vi "Day12-validate_path_2.vi"(11 "Path":string[](array[string])) -> (1 "invalid?":bool, 2 "finshed?":bool, 3 "Path out":string[](array[string]))   [LabVIEW 2021]
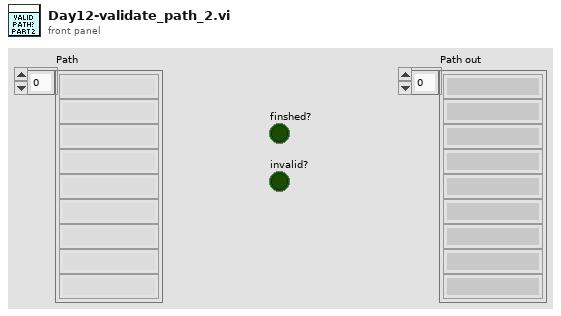
[diagram p1: front panel]
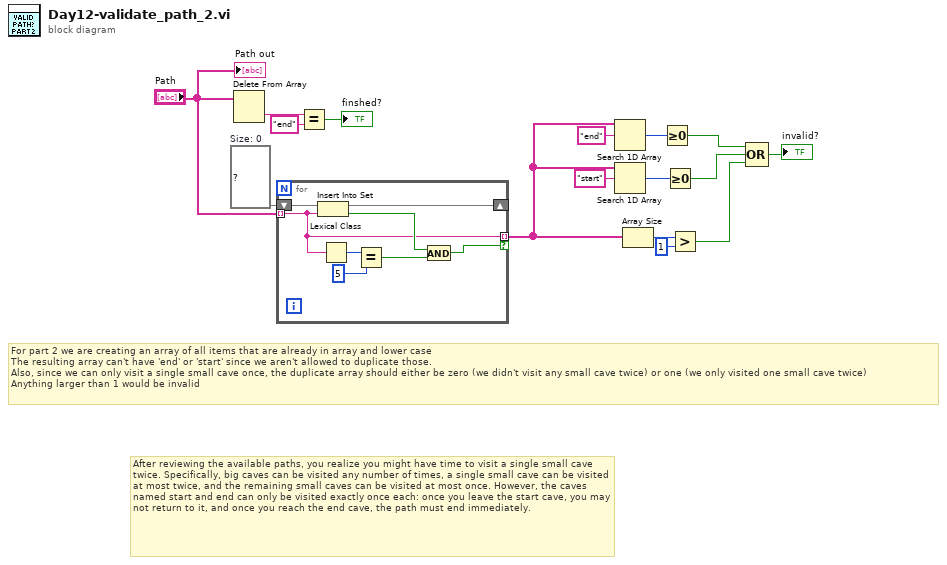
[diagram p0: block diagram]
diagram:
  w13 = set{string} {}  # Size: 0
  # "After reviewing the available paths, you realize you might have time to visit a single small cave twice. Specifically, big caves can be visited any number of times, a single small cave can be visited at most twice, and the remaining small caves can be visited at most once. However, the caves named start and end can only be visited exactly once each: once you leave the start cave, you may not return to it, and once you reach the end cave, the path must end immediately."
  # "For part 2 we are creating an array of all items that are already in array and lower case\nThe resulting array can't have 'end' or 'start' since we aren't allowed to duplicate those.\nAlso, since we can only visit a single small cave once, the duplicate array should either be zero (we didn't visit any small cave twice) or one (we only visited one small cave twice)\nAnything larger than 1 would be invalid"
  n1 = Delete From Array(array="Path") -> (deleted portion=w16:string)  [unwired: 2 in, 1 out]
  n2 = for {
    tunnel: "Path" -> [w18] mode=indexing
    shift-right: [w24] -> _
    shift-left: w13 -> [w23]
    tunnel: [w18] -> w4 mode=indexing if=w17
    n3 = Insert Into Set(10:w18, 11:w23) -> (2:w20:bool, 3:w24:set{string})
    n4 = Lexical Class(1:w18) -> (0:w22:i16)
    n5 = Equal?(x=w22, y=i16 5) -> (x = y?=w19:bool)
    n6 = And(x=w20, y=w19) -> (x .and. y?=w17:bool)
  }
  n7 = Equal?(x=w16, y="end") -> (x = y?=→"finshed?":bool)
  n8 = Search 1D Array(1D array=w4, element="end") -> (index of element=w9:i32)  [unwired: 1 in]
  n9 = Search 1D Array(1D array=w4, element="start") -> (index of element=w8:i32)  [unwired: 1 in]
  n10 = Array Size(array=w4) -> (size(s)=w3:i32)
  n11 = Greater Or Equal To 0?(x=w9) -> (x >= 0?=w7:bool)
  n12 = Greater Or Equal To 0?(x=w8) -> (x >= 0?=w6:bool)
  n13 = Greater?(x=w3, y=1) -> (0:w1:bool)
  n14 = Compound Arithmetic op=OR(w7, w6, w1) -> (→"invalid?":bool)
  "Path out" <- "Path"
